vi "HexStringToU8Array.vi"(11 "HEX String (0-9,A-F)":string) -> (3 "u8 Data[]":u8[](array[numeric]) format="%.0x")   [LabVIEW 2015]
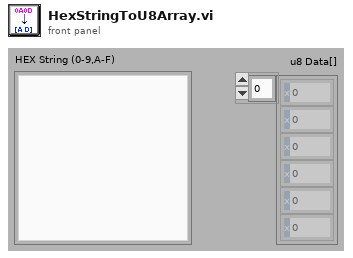
[diagram p1: front panel]
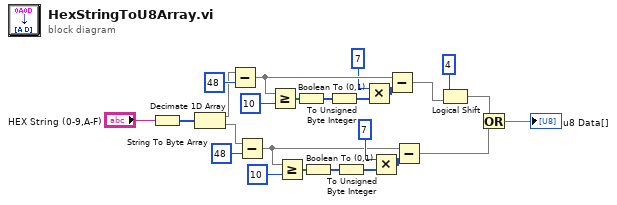
[diagram p0: block diagram]
diagram:
  n1 = String To Byte Array(string="HEX String (0-9,A-F)") -> (unsigned byte array=w23:u8[])
  n2 = Decimate 1D Array(w23) -> (w1:u8[], w21:u8[])
  n3 = Subtract(x=w1, y=u8 48) -> (x-y=w9:u8[])
  n4 = Subtract(x=w21, y=u8 48) -> (x-y=w13:u8[])
  n5 = Greater Or Equal?(x=w9, y=u8 10) -> (x >= y?=w6:bool[])
  n6 = Greater Or Equal?(x=w13, y=u8 10) -> (x >= y?=w16:bool[])
  n7 = Boolean To (0,1)(Boolean=w6) -> (0, 1=w4:i16[])
  n8 = Boolean To (0,1)(Boolean=w16) -> (0, 1=w18:i16[])
  n9 = To Unsigned Byte Integer(number=w4) -> (unsigned 8bit integer=w7:u8[])
  n10 = To Unsigned Byte Integer(number=w18) -> (unsigned 8bit integer=w15:u8[])
  n11 = Multiply(x=u8 7, y=w7) -> (x*y=w8:u8[])
  n12 = Multiply(x=u8 7, y=w15) -> (x*y=w14:u8[])
  n13 = Subtract(x=w9, y=w8) -> (x-y=w10:u8[])
  n14 = Subtract(x=w13, y=w14) -> (x-y=w22:u8[])
  n15 = Logical Shift(y=i8 4, x=w10) -> (x << y=w12:u8[])
  n16 = Or(x=w12, y=w22) -> (x .or. y?=→"u8 Data[]":u8[])
